vi "Close.vi"(8 "error in":errorcluster, 11 "Current Control in":refnum<class "Current Control.lvclass">) -> (0 "error out":errorcluster, 3 "Current Control out":refnum<class "Current Control.lvclass">)   [LabVIEW 2023, in "Current Control.lvclass"]
uses:
  Current Control.lvclass
  Current Control.lvclass/Current Control.ctl
  <vilib>/ADAS Replay HIL/AdasHilServices/AdasHilServices Fill In Error Info Ex.vi
  <vilib>/ADAS Replay HIL/AdasHilServices/AdasHilChannelServices.lvlib
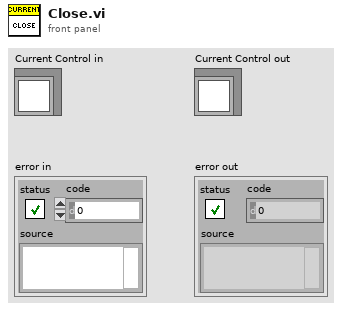
[diagram p1: front panel]
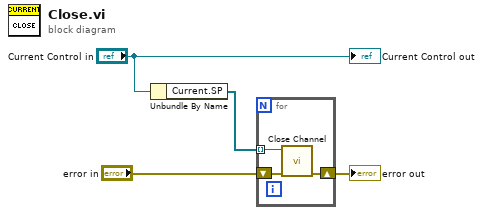
[diagram p0: block diagram]
diagram:
  n1 = Unbundle By Name("Current Control in") -> ("Current.SP"=w2:refnum<k21>[])
  n2 = for {
    tunnel: w2 -> [w5] mode=indexing
    shift-right: [w7] -> w4
    shift-left: "error in" -> [w6]
    n3 = call <vilib>:"Close Channel.vi"("error in"=w6, "ADAS HIL Channel"=w5) -> ("error out"=w7:errorcluster)  [unwired: 9 in]
  }
  "error out" <- w4
  "Current Control out" <- "Current Control in"
